vi "test.vi"() -> ()   [LabVIEW 2016]
panel:
  out "Waveform Graph":sgl[][](graph)
  out "Numeric":i32
  in  "Array 2":dbl[](array[numeric]) format="%#_13g"
  in  "Interval(mV/uA)":dbl format="%#_13g"
  in  "Compliance  Level (A/V)":dbl=0.1
  in  "Array":dbl[](array[numeric]) format="%#_13g"
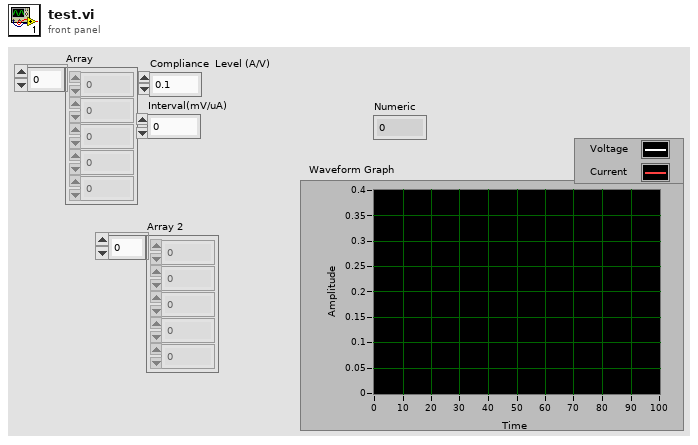
[diagram p1: front panel]
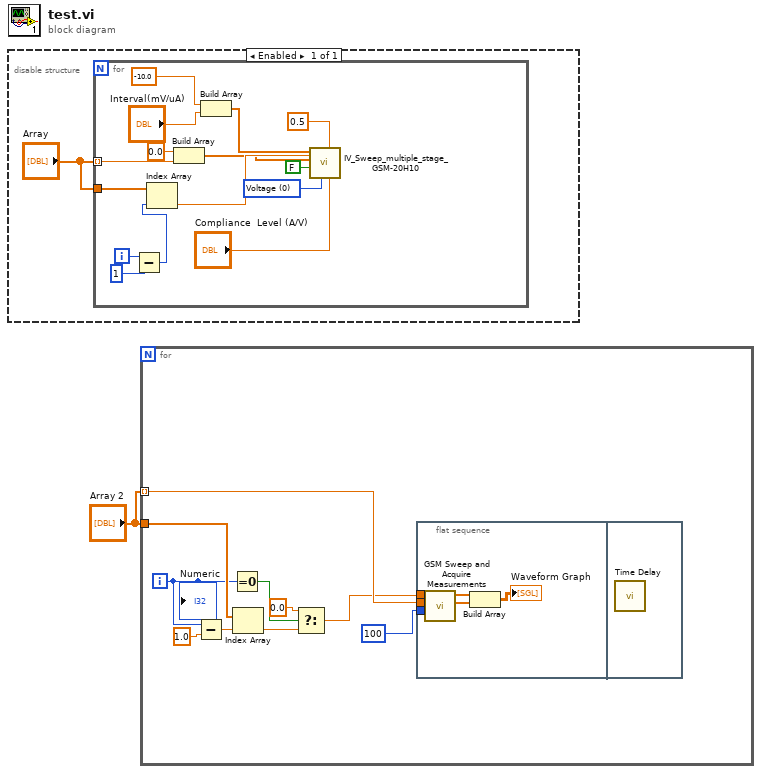
[diagram p0: block diagram]
diagram:
  n1 = disable-structure shown="Enabled" {
    frame Enabled {
      n2 = for {
        tunnel: "Array" -> [w5] mode=indexing
        tunnel: "Array" -> [w17]
        i -> [w16]
        w12 = u16 0 items=["Voltage", "Current"] ("Source Mode  (0: Voltage)")
        n3 = Subtract(x=w16, y=1) -> (x-y=w14:i32)
        n4 = Index Array(array=w17, index=w14) -> (element=w7:dbl)
        n5 = Build Array(0.0 ("element"), w5) -> (w6:dbl[])
        n6 = Build Array(-10.0 ("element"), "Interval(mV/uA)") -> (w9:dbl[])
        n7 = call "IV_Sweep_multiple_stage_GSM-20H10.vi"("Compliance  Level (A/V)"="Compliance  Level (A/V)", "Delay Time (s)"=0.5, "Source Mode  (0: Voltage)"=w12, "End (mV/uA)"=w7, "Writefile"=FALSE, "Start(V/mA)"=w6, "Interval (mV/uA)"=w9) -> ()  [unwired: 2 in, 3 out]
      }
    }
  }
  n8 = for {
    tunnel: "Array 2" -> [w27] mode=indexing
    tunnel: "Array 2" -> [w23]
    i -> [w21]
    n9 = Subtract(x=w21, y=1.0) -> (x-y=w20:dbl)
    n10 = Equal To 0?(x=w21) -> (x = 0?=w26:bool)
    n11 = Index Array(array=w23, index=w20) -> (element=w24:dbl)
    n12 = Select(t=0.0, s=w26, f=w24) -> (s? t:f=w19:dbl)
    n13 = flat-sequence {
      tunnel: w27 -> [w33]
      tunnel: w19 -> [w32]
      tunnel: u32 100 ("Number of Points (5)") -> [w31]
      frame #0 {
        n14 = call <instrlib>:"GSM Sweep and Acquire Measurements.vi"("Number of Points (5)"=w31, "Maximum Amplitude (2)"=w33, "Minimum Amplitude (1)"=w32) -> ("Current"=w29:sgl[], "Voltage"=w30:sgl[])  [unwired: 4 in, 1 out]
        n15 = Build Array(w30, w29) -> (→"Waveform Graph":sgl[][])
      }
      frame #1 {
        n16 = call "Time Delay"() -> ()  [unwired: 11 in, 1 out]
      }
    }
    "Numeric" <- w21
  }
